vi "Polarization_Simulation.vi"() -> ()   [LabVIEW 2018]
panel:
  in  "Drive Zero Level Down":bool
  in  "Thermally Connect Zero Ensemble":bool
  in  "Zero Ensemble Power":dbl=0.05
  in  "Zero Lorentzian Position":dbl=1.0
  in  "Zero Lorentzian Width":dbl=0.05
  in  "Zero Ensemble Area":dbl=0.1
  in  "Zero Level on":bool
  in  "Gaussian Noise SD":dbl
  in  "AFP Efficiency":dbl=0.8
  in  "Timing (ms)":i32=10
  out "XY Graph 3":cluster{dbl[], "rho- out":dbl[]}[](graph)
  in  "AFP Sweep Direction":u16(ring) items=["Positive", "Negative"]
  in  "RF Proportional to Intensity":bool
  in  "File operation":u16(ring) items=["Open existing file", "Create new file", "Replace existing file"]
  out "XY Graph 2":cluster{"Array":dbl[], "Array 2":dbl[]}(graph)
  in  "Sweep AFP Range":bool
  in  "RF Power":dbl=0.1 min=0.0 max=1.0 step=0.01
  in  "Also use RF Range 2":bool
  in  "RF on":bool
  out "XY Graph":cluster{dbl[], "rho+ array out":dbl[]}[](graph)
  in  "Microwave on":bool
  in  "AFP Slider":cluster{i32, i32}(slide)={0, 500} scale=0.0..500.0
  in  "RF Slider 2":cluster{i32, i32}(slide)={0, 4} scale=0.0..500.0
  in  "RF Slider 1":cluster{i32, i32}(slide)={201, 238} scale=0.0..500.0
  in  "Relaxation Rate":dbl min=0.0 max=1.0 step=0.0001
  in  "Microwave Power":dbl=0.05 min=0.0 max=1.0 step=0.001
  in  "Saturation Polarization":dbl=0.45 min=0.0 max=0.99 step=0.01
  in  "Signal Lorentzian Width":dbl=0.005 min=0.0 step=0.001
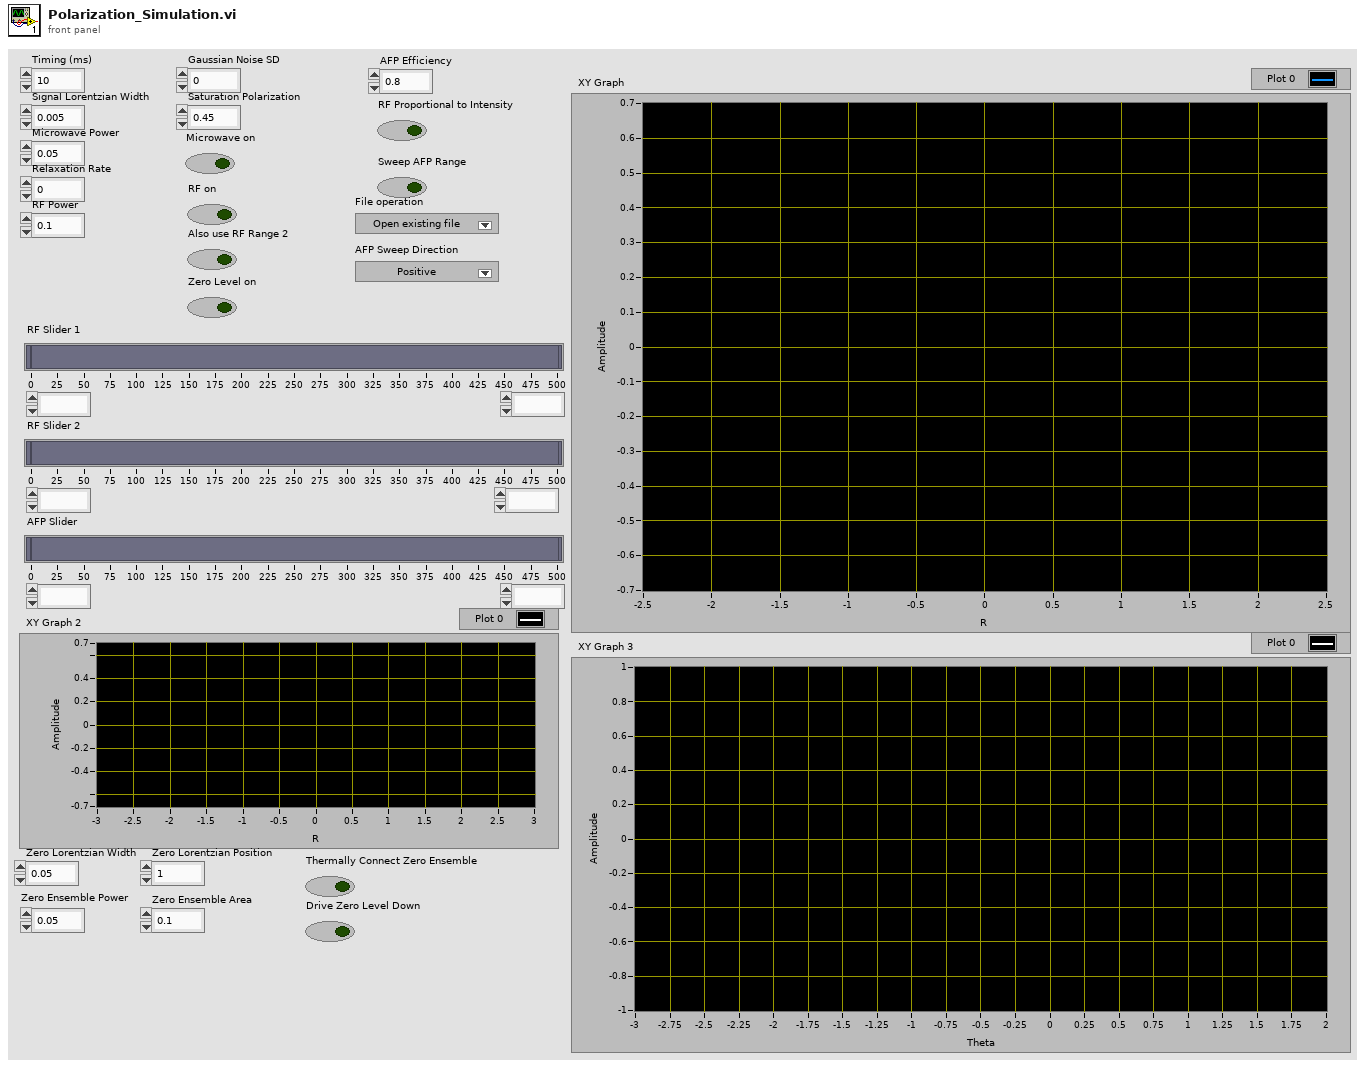
[diagram p1: front panel]
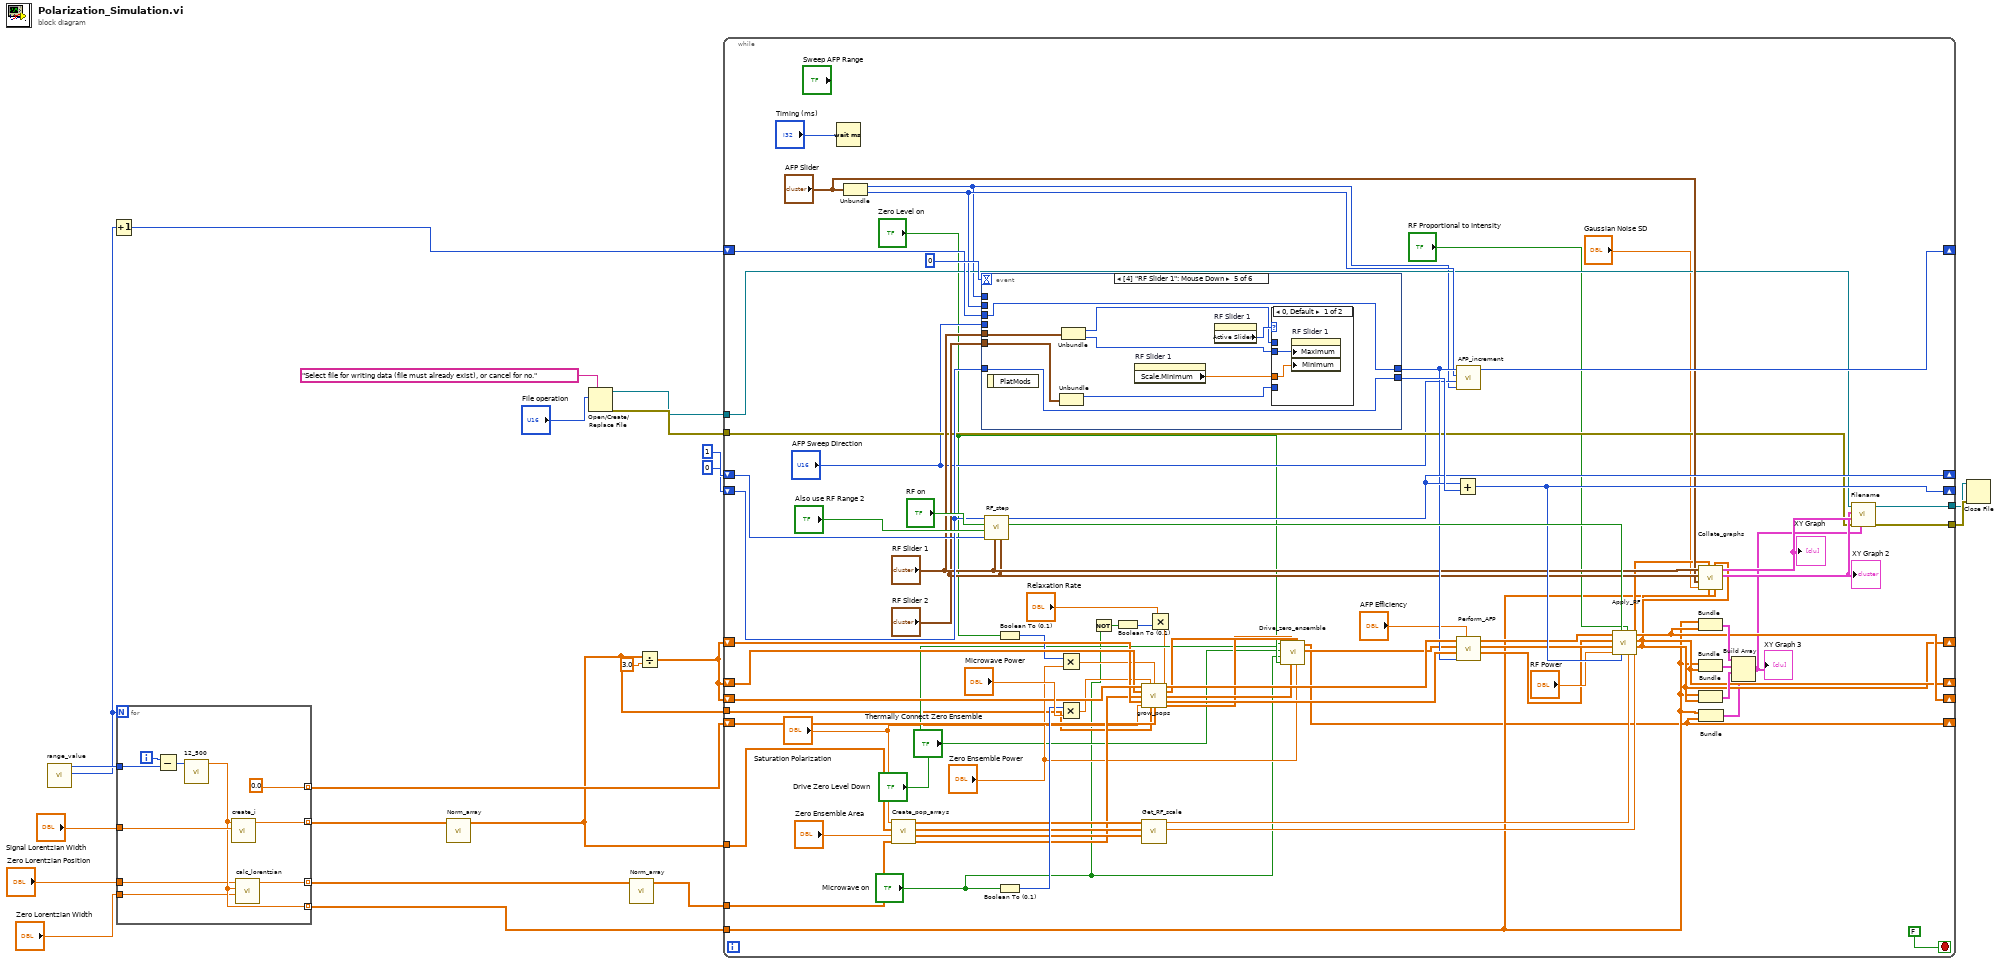
[diagram p0: block diagram]
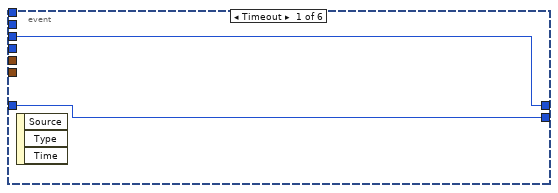
[diagram p2: hidden frame]
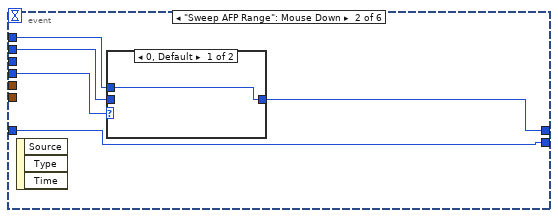
[diagram p3: hidden frame]
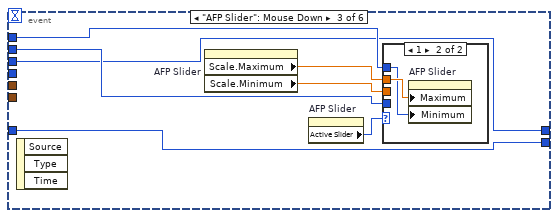
[diagram p5: hidden frame]
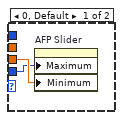
[diagram p6: hidden frame]
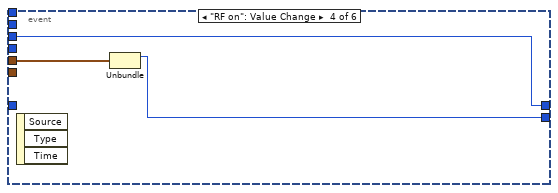
[diagram p7: hidden frame]
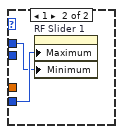
[diagram p8: hidden frame]
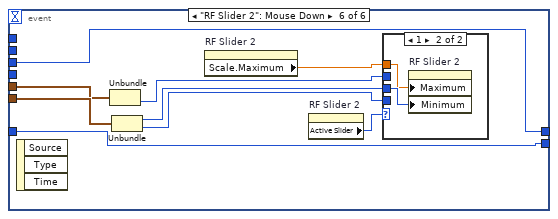
[diagram p9: hidden frame]
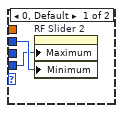
[diagram p10: hidden frame]
diagram:
  n1 = call "range_value.vi"() -> ("NumBins"=w16:i32, "Center"=w22:i32)  [unwired: 10 in]
  n2 = Increment(x=w16) -> (x+1=w15:i32)
  n3 = for {
    N: w16 -> [_]
    tunnel: [w30] -> w20 mode=indexing
    tunnel: w22 -> [w29]
    tunnel: "Signal Lorentzian Width" -> [w28]
    tunnel: [w26] -> w19 mode=indexing
    tunnel: [w27] -> w6 mode=indexing
    tunnel: "Zero Lorentzian Width" -> [w25]
    tunnel: "Zero Lorentzian Position" -> [w24]
    tunnel: [0.0] -> w2 mode=indexing
    i -> [w32]
    n4 = Subtract(x=w32, y=w29) -> (x-y=w31:i32)
    n5 = call "12_500.vi"("Numeric in"=w31) -> ("Numeric out"=w26:dbl)  [unwired: 10 in]
    n6 = call "create_i.vi"("Lorentzian Width"=w28, "Numeric"=w26) -> ("Numeric 2"=w30:dbl)  [unwired: 9 in]
    n7 = call "calc_lorentzian.vi"("Width in"=w25, "x in"=w26, "Position in"=w24) -> ("Value out"=w27:dbl)  [unwired: 8 in]
  }
  n8 = call "Norm_array.vi"("Array"=w20) -> ("Normed Array"=w1:dbl[])  [unwired: 10 in]
  n9 = Open/Create/Replace File(prompt="Select file for writing data (file must already exist), or cancel for no.", operation (0:open)="File operation") -> (refnum out=w12:refnum<file>, error out=w14:errorcluster)  [unwired: 4 in, 1 out]
  n10 = call "Norm_array.vi"("Array"=w6) -> ("Normed Array"=w3:dbl[])  [unwired: 10 in]
  n11 = Divide(x=w1, y=3.0) -> (x/y=w7:dbl[])
  n12 = while {
    tunnel: w1 -> [w109]
    shift-right: [w65] -> _
    shift-left: w7 -> [w106]
    shift-right: [w63] -> _
    shift-left: w7 -> [w104]
    shift-right: [w64] -> _
    shift-left: w7 -> [w105]
    tunnel: w19 -> [w42]
    shift-right: [w94] -> _
    shift-left: 1 -> [w92]
    shift-right: [w96] -> _
    shift-left: 0 -> [w93]
    shift-right: [w90] -> _
    shift-left: w15 -> [w91]
    tunnel: w14 -> [w80]
    tunnel: [w79] -> w13
    tunnel: w12 -> [w78]
    tunnel: [w77] -> w11
    tunnel: w3 -> [w55]
    shift-right: [w41] -> _
    shift-left: w2 -> [w51]
    tunnel: w1 -> [w37]
    stop <- FALSE stop-if-true
    n13 = Wait (ms)(milliseconds to wait="Timing (ms)") -> ()  [unwired: 1 out]
    n14 = Unbundle("AFP Slider") -> (w69:i32, w86:i32)
    n15 = call "Create_pop_arrays.vi"("Zero ensemble in"=w55, "Zero ensemble area in"="Zero Ensemble Area", "Normalized I in"=w109, "Saturation Polarization"="Saturation Polarization") -> ("Zero ensemble out"=w54:dbl[], "rho- array out"=w74:dbl[], "rho0 array out"=w75:dbl[], "rho+ array out"=w76:dbl[])  [unwired: 4 in]
    n16 = event shown="[4] \"RF Slider 1\": Mouse Down" {
      selector: _ -> [_ _ _ _ _ _]
      dyn-events: _ -> [_ _ _ _ _ _]
      timeout: 0 -> [_ _ _ _ _ _]
      tunnel: "RF Slider 2" -> [_ _ _ _ w137 w155]
      tunnel: "RF Slider 1" -> [_ _ _ w133 w138 w154]
      tunnel: [w112 w117 w120 w132 w135 w148] -> w97
      tunnel: w93 -> [w112 w117 w120 _ w135 w148]
      tunnel: [w111 w114 w121 w131 w134 w147] -> w87
      tunnel: w91 -> [w111 _ w121 w131 w134 w147]
      tunnel: w69 -> [_ w113 w123 _ _ _]
      tunnel: w86 -> [_ w115 w122 _ _ _]
      tunnel: "AFP Sweep Direction" -> [_ w116 _ _ _ _]
      event Timeout {
        n17 = event-data() -> ()  [unwired: 1 in, 3 out]
      }
      event "Sweep AFP Range": Mouse Down {
        n18 = event-data() -> ()  [unwired: 1 in, 3 out]
        n19 = case shown="0, Default" w116 {
          tunnel: [w118 w119] -> w114
          tunnel: w115 -> [_ w119]
          tunnel: w113 -> [w118 _]
          frame 0, Default {
          }
          frame 1 {
          }
        }
      }
      event "AFP Slider": Mouse Down {
        n20 = event-data() -> ()  [unwired: 1 in, 3 out]
        n21 = property on="AFP Slider" class="Slide (strict)"() -> ("Scale.Maximum"=w125:dbl, "Scale.Minimum"=w124:dbl)  [unwired: 2 in, 2 out]
        n22 = property on="AFP Slider" class="Slide (strict)"() -> ("Active Slider"=w126:i32)  [unwired: 2 in, 2 out]
        n23 = case shown="1" w126 {
          tunnel: w125 -> [_ w130]
          tunnel: w124 -> [w128 _]
          tunnel: w123 -> [_ w129]
          tunnel: w122 -> [w127 _]
          frame 0, Default {
            n24 = property on="AFP Slider" class="Slide (strict)"("Maximum"=w127, "Minimum"=w128) -> ()  [unwired: 2 in, 2 out]
          }
          frame 1 {
            n25 = property on="AFP Slider" class="Slide (strict)"("Maximum"=w130, "Minimum"=w129) -> ()  [unwired: 2 in, 2 out]
          }
        }
      }
      event "RF on": Value Change {
        n26 = event-data() -> ()  [unwired: 1 in, 3 out]
        n27 = Unbundle(w133) -> (w132:i32)  [unwired: 1 out]
      }
      event "RF Slider 1": Mouse Down {
        n28 = event-data() -> ()  [unwired: 1 in, 1 out]
        n29 = Unbundle(w137) -> (w136:i32)  [unwired: 1 out]
        n30 = Unbundle(w138) -> (w141:i32, w140:i32)
        n31 = property on="RF Slider 1" class="Slide (strict)"() -> ("Scale.Minimum"=w139:dbl)  [unwired: 2 in, 2 out]
        n32 = property on="RF Slider 1" class="Slide (strict)"() -> ("Active Slider"=w142:i32)  [unwired: 2 in, 2 out]
        n33 = case shown="0, Default" w142 {
          tunnel: w136 -> [_ w146]
          tunnel: w141 -> [_ w145]
          tunnel: w140 -> [w144 _]
          tunnel: w139 -> [w143 _]
          frame 0, Default {
            n34 = property on="RF Slider 1" class="Slide (strict)"("Maximum"=w144, "Minimum"=w143) -> ()  [unwired: 2 in, 2 out]
          }
          frame 1 {
            n35 = property on="RF Slider 1" class="Slide (strict)"("Maximum"=w146, "Minimum"=w145) -> ()  [unwired: 2 in, 2 out]
          }
        }
      }
      event "RF Slider 2": Mouse Down {
        n36 = event-data() -> ()  [unwired: 1 in, 3 out]
        n37 = Unbundle(w154) -> (w152:i32)  [unwired: 1 out]
        n38 = Unbundle(w155) -> (w150:i32, w151:i32)
        n39 = property on="RF Slider 2" class="Slide (strict)"() -> ("Scale.Maximum"=w149:dbl)  [unwired: 2 in, 2 out]
        n40 = property on="RF Slider 2" class="Slide (strict)"() -> ("Active Slider"=w153:i32)  [unwired: 2 in, 2 out]
        n41 = case shown="1" w153 {
          tunnel: w152 -> [w157 _]
          tunnel: w151 -> [w156 _]
          tunnel: w150 -> [_ w159]
          tunnel: w149 -> [_ w158]
          frame 0, Default {
            n42 = property on="RF Slider 2" class="Slide (strict)"("Maximum"=w156, "Minimum"=w157) -> ()  [unwired: 2 in, 2 out]
          }
          frame 1 {
            n43 = property on="RF Slider 2" class="Slide (strict)"("Maximum"=w158, "Minimum"=w159) -> ()  [unwired: 2 in, 2 out]
          }
        }
      }
    }
    n44 = call "RF_step.vi"("RF Range 2"="RF Slider 2", "RF Range 1"="RF Slider 1", "RF Step Value"=w92, "2 ranges?"="Also use RF Range 2", "RF on"="RF on", "RF Location"=w93) -> ("RF Indicator"=w98:bool, "RF Location out"=w94:i32)  [unwired: 4 in]
    n45 = Boolean To (0,1)(Boolean="Zero Level on") -> (0, 1=w53:i16)
    n46 = Boolean To (0,1)(Boolean="Microwave on") -> (0, 1=w102:i16)
    n47 = Multiply(x=w53, y="Zero Ensemble Power") -> (x*y=w52:dbl)
    n48 = Multiply(x=w102, y="Microwave Power") -> (x*y=w103:dbl)
    n49 = Not(x="Microwave on") -> (.not. x?=w34:bool)
    n50 = Boolean To (0,1)(Boolean=w34) -> (0, 1=w35:i16)
    n51 = call "Get_RF_scale.vi"("rho-"=w74, "rho0"=w75, "rho+"=w76) -> ("I-  index out"=w72:dbl, "I+ index out"=w73:dbl)  [unwired: 7 in]
    n52 = Multiply(x="Relaxation Rate", y=w35) -> (x*y=w36:dbl)
    n53 = call "grow_pops.vi"("rho+ array"=w106, "Microwave power"=w103, "Zero Level Power"=w52, "Decay rate"=w36, "rho0 array"=w105, "Zero Ensemble Condition"=w54, "rho- array"=w104, "Sat pol"="Saturation Polarization", "I array"=w37, "Zero Ensemble Array"=w51) -> ("rho+ array out"=w88:dbl[], "rho0 array out"=w50:dbl[], "rho0 decay out"=w49:dbl[], "rho- array out"=w89:dbl[], "Zero Ensemble Out"=w48:dbl[])  [unwired: 1 in]
    n54 = call "Drive_zero_ensemble.vi"("Zero ensemble power in"="Zero Ensemble Power", "rho0 in"=w50, "rho0 decay in"=w49, "Zero ensemble in"=w48, "Drive Zero Ensemble Up"="Zero Level on", "Microwave on"="Microwave on", "Drive Zero Ensemble Down"="Drive Zero Level Down", "Thermal connection"="Thermally Connect Zero Ensemble") -> ("rho0 out"=w47:dbl[], "Zero ensemble out"=w41:dbl[])  [unwired: 2 in]
    n55 = Add(x=w94, y=w97) -> (x+y=w96:i32)
    n56 = call "AFP_increment.vi"("AFP Min"=w69, "Sweep Direction"="AFP Sweep Direction", "AFP Max"=w86, "AFP Target"=w87) -> ("AFP Target Out"=w90:i32)  [unwired: 7 in]
    n57 = call "Perform_AFP.vi"("AFP Efficiency"="AFP Efficiency", "AFP Target"=w87, "rho-"=w89, "rho0"=w47, "rho+"=w88) -> ("rho- out"=w57:dbl[], "rho0 out"=w58:dbl[], "rho+ out"=w59:dbl[])  [unwired: 4 in]
    n58 = call "Apply_RF.vi"("I- index"=w72, "I+ index"=w73, "RF Proportional to intensity"="RF Proportional to Intensity", "RF Target Position"=w96, "RF indicator"=w98, "RF Power"="RF Power", "rho0"=w58, "rho-"=w57, "rho+"=w59) -> ("rho- out"=w63:dbl[], "rho0 out"=w64:dbl[], "rho+ out"=w65:dbl[])
    n59 = call "Collate_graphs.vi"("R values"=w42, "rho0"=w64, "rho-"=w63, "rho+"=w65, "Gaussian SD in"="Gaussian Noise SD", "AFP Range"="AFP Slider", "RF Range 2"="RF Slider 2", "RF Range 1"="RF Slider 1") -> ("Q Graph"=w81:cluster{"Array":dbl[], "Array 2":dbl[]}, "P Graph and Intensities and RF"=w82:cluster{"Array":dbl[], "Array":dbl[]}[])  [unwired: 2 in]
    "XY Graph" <- w82
    "XY Graph 2" <- w81
    n60 = Bundle(w42, "rho+ out"=w65) -> (w67:cluster{dbl[], "rho+ out":dbl[]})  [unwired: 1 in]
    n61 = Bundle(w42, "rho0 out"=w64) -> (w68:cluster{dbl[], "rho0 out":dbl[]})  [unwired: 1 in]
    n62 = Bundle(w42, "rho- out"=w63) -> (w66:cluster{dbl[], "rho- out":dbl[]})  [unwired: 1 in]
    n63 = Bundle(w42, "Zero ensemble out"=w41) -> (w40:cluster{dbl[], "Zero ensemble out":dbl[]})  [unwired: 1 in]
    n64 = Build Array(w67, w68, w66, w40) -> (w39:cluster{dbl[], "Zero ensemble out":dbl[]}[])
    "XY Graph 3" <- w39
    n65 = call "Filename.vi"("Densities and De Boer"=w39, "error in (no error)"=w80, "P Graph and Intensities and RF"=w82, "Q Graph"=w81, "Byte Stream File in"=w78) -> ("error out"=w79:errorcluster, "Byte Stream File out"=w77:refnum<file>)  [unwired: 5 in]
  }
  n66 = Close File(refnum=w11, error in=w13) -> ()  [unwired: 2 out]
